vi "Ini_LogFile.vi"() -> (0 "error out":errorcluster, 3 "logFile Path":refnum<file>)   [LabVIEW 2018]
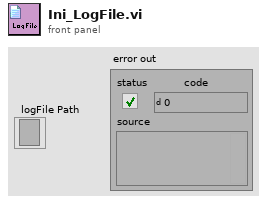
[diagram p1: front panel]
types:
  T1 = enum16{"open", "replace", "create", "open or create", "replace or create", "replace or create with confirmation"}
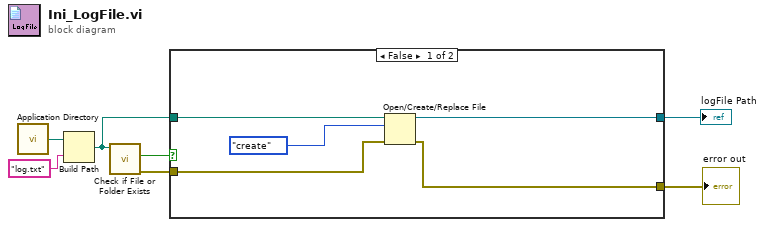
[diagram p0: block diagram]
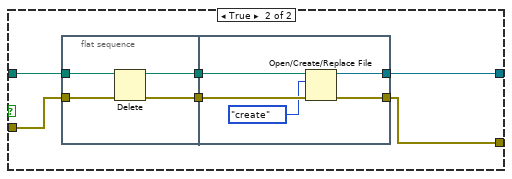
[diagram p2: hidden frame]
diagram:
  n1 = call <vilib>:"Application Directory.vi"() -> ("Application Directory"=w3:path)
  n2 = Build Path(base path=w3, name or relative path="log.txt") -> (appended path=w6:path)
  n3 = call <vilib>:"Check if File or Folder Exists.vi"("path"=w6) -> ("error out"=w7:errorcluster, "file or folder exists?"=w5:bool)  [unwired: 8 in, 1 out]
  n4 = case shown="False" w5 {
    tunnel: w6 -> [w12 w18]
    tunnel: w7 -> [w11 w17]
    tunnel: [w9 w14] -> w2
    tunnel: [w8 w13] -> w1
    frame False {
      n5 = Open/Create/Replace File(file path (use dialog)=w12, error in=w11, operation (0:open)=T1."create") -> (refnum out=w9:refnum<file>, error out=w8:errorcluster)  [unwired: 3 in, 1 out]
    }
    frame True {
      n6 = flat-sequence {
        tunnel: w18 -> [w22]
        tunnel: w17 -> [w21]
        tunnel: [w20] -> w16
        tunnel: [w19] -> w15
        tunnel: w16 -> [w27]
        tunnel: w15 -> [w26]
        tunnel: [w24] -> w14
        tunnel: [w23] -> w13
        frame #0 {
          n7 = Delete(path (use dialog)=w22, error in=w21) -> (deleted path=w19:path, error out=w20:errorcluster)  [unwired: 3 in, 1 out]
        }
        frame #1 {
          n8 = Open/Create/Replace File(file path (use dialog)=w26, error in=w27, operation (0:open)=T1."create") -> (refnum out=w24:refnum<file>, error out=w23:errorcluster)  [unwired: 3 in, 1 out]
        }
      }
    }
  }
  "logFile Path" <- w2
  "error out" <- w1
